vi "set channel.vi"(0 "VISA in":refnum<visa-resource-name>, 1 "Location Cluster in":T1, 2 "set row":i32, 3 "set card":i32, 4 "set channel":i32, 5 "error in":errorcluster) -> (14 "VISA out":refnum<visa-resource-name>, 15 "Location Cluster out":T1, 19 "error out":errorcluster)   [LabVIEW 2018]
uses:
  location cluster.ctl
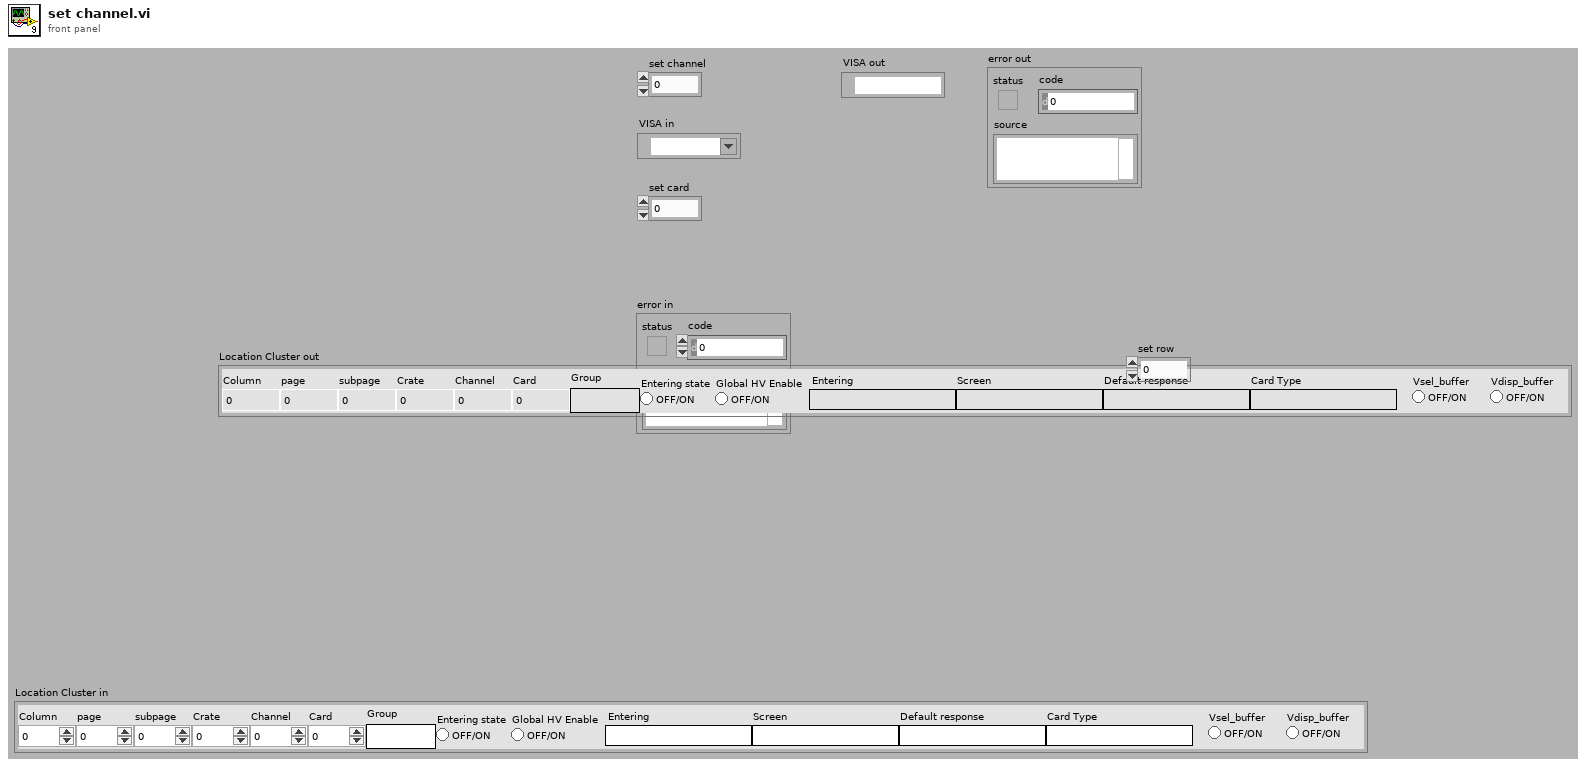
[diagram p1: front panel]
types:
  T1 = typedef "location cluster.ctl" = cluster{"Column":i32, "Card Type":string, "Channel":i32, "Card":i32, "Default response":string, "Entering":string, "Entering state":bool, "subpage":i32, "page":i32, "Crate":i32, "Screen":string, "Group":string, "Global HV Enable":bool, "Vsel_buffer":bool, "Vdisp_buffer":bool}
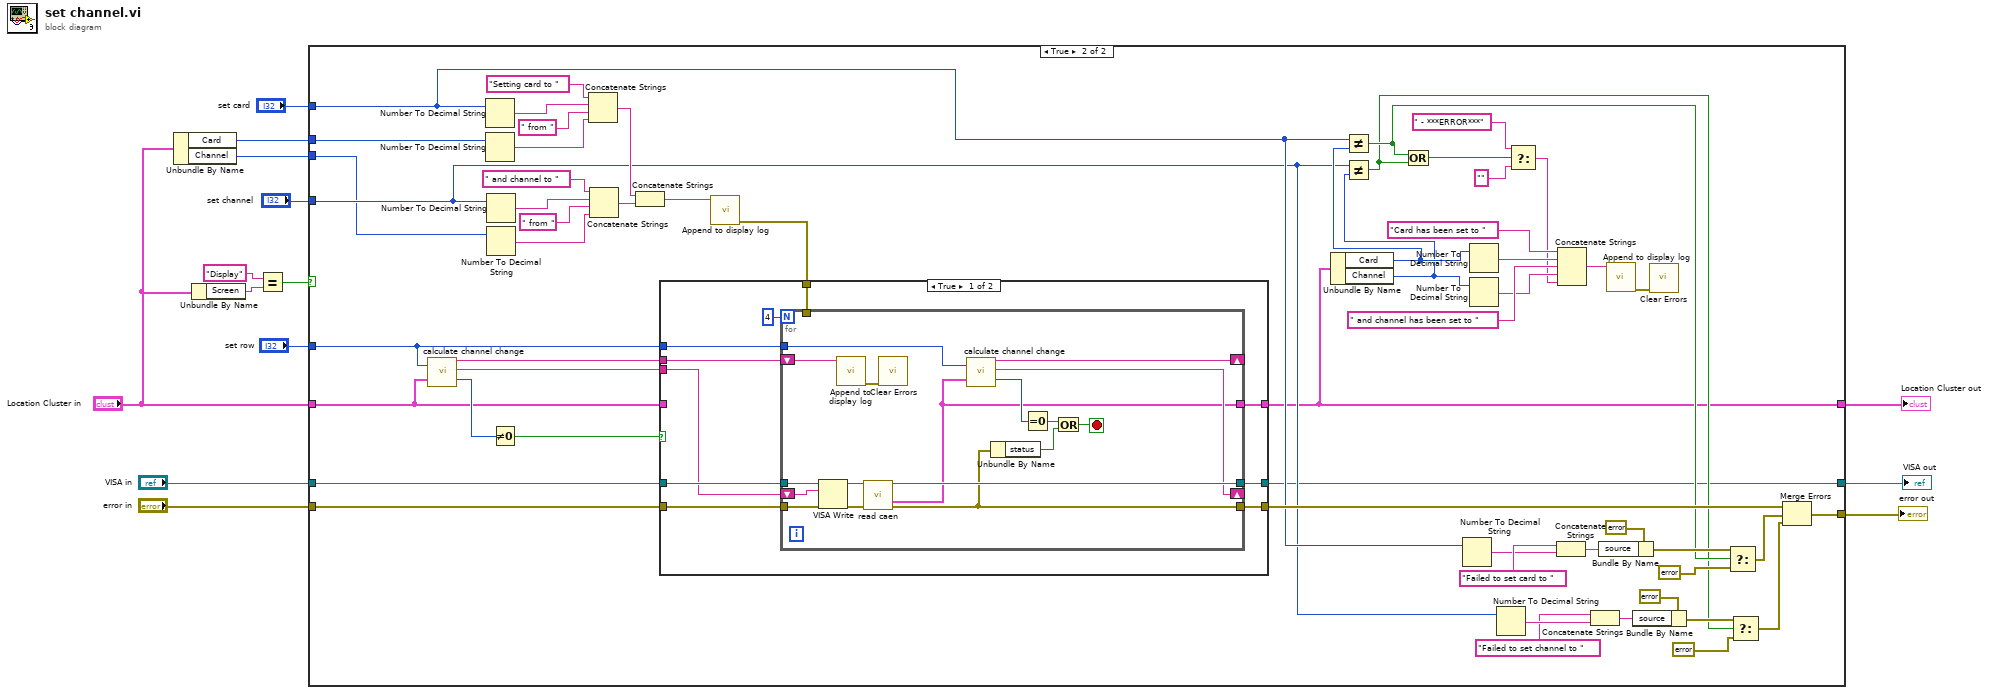
[diagram p0: block diagram]
diagram:
  n1 = Unbundle By Name("Location Cluster in") -> ("Card"=w9:i32, "Channel"=w2:i32)
  n2 = Unbundle By Name("Location Cluster in") -> ("Screen"=w12:string)
  n3 = Equal?(x="Display", y=w12) -> (x = y?=w5:bool)
  n4 = case shown="True" w5 {
    tunnel: "VISA in" -> [w16 w73]
    tunnel: "Location Cluster in" -> [w15 w18]
    tunnel: "error in" -> [w17 w19]
    tunnel: w9 -> [_ w48]
    tunnel: [w17 w36] -> w8
    tunnel: "set card" -> [_ w26]
    tunnel: "set channel" -> [_ w25]
    tunnel: w2 -> [_ w24]
    tunnel: [w15 w22] -> w4
    tunnel: [w16 w21] -> w3
    tunnel: "set row" -> [_ w20]
    frame False {
    }
    frame True {
      n5 = call "calculate channel change.vi"("set index"=w20, "Location Cluster in"=w18) -> ("action"=w46:string, "keystrokes"=w47:string, "rows difference"=w45:i32)  [unwired: 15 in]
      n6 = Number To Decimal String(number=w26) -> (decimal integer string=w66:string)  [unwired: 1 in]
      n7 = Number To Decimal String(number=w48) -> (decimal integer string=w68:string)  [unwired: 1 in]
      n8 = Number To Decimal String(number=w25) -> (decimal integer string=w71:string)  [unwired: 1 in]
      n9 = Number To Decimal String(number=w24) -> (decimal integer string=w69:string)  [unwired: 1 in]
      n10 = Not Equal To 0?(x=w45) -> (x != 0?=w23:bool)
      n11 = Concatenate Strings("Setting card to " ("string"), w66, " from " ("string"), w68) -> (w64:string)
      n12 = Concatenate Strings(" and channel to " ("string"), w71, " from " ("string"), w69) -> (w63:string)
      n13 = Concatenate Strings(w64, w63) -> (w62:string)
      n14 = call "Append to display log.vi"("string"=w62) -> ("error out"=w61:errorcluster)  [unwired: 10 in]
      n15 = case shown="True" w23 {
        tunnel: [w76 w103] -> w21
        tunnel: w73 -> [w83 w103]
        tunnel: [w82 w102] -> w37
        tunnel: w19 -> [w81 w102]
        tunnel: [w77 w101] -> w22
        tunnel: w18 -> [_ w101]
        tunnel: w61 -> [w74 _]
        tunnel: w20 -> [w80 _]
        tunnel: w47 -> [w78 _]
        tunnel: w46 -> [w79 _]
        frame True {
          n16 = for {
            N: 4 -> [_]
            tunnel: w80 -> [w95]
            tunnel: [w84] -> w77
            shift-right: [w86] -> _
            shift-left: w78 -> [w93]
            shift-right: [w85] -> _
            shift-left: w79 -> [w94]
            tunnel: w83 -> [w100]
            tunnel: [w91] -> w76
            tunnel: w81 -> [w97]
            tunnel: [w90] -> w82
            tunnel: w74 -> [_]
            stop <- w87 stop-if-true
            n17 = VISA Write(VISA resource name=w100, write buffer=w93, error in (no error)=w97) -> (VISA resource name out=w99:refnum<visa-resource-name>, error out=w98:errorcluster)  [unwired: 1 out]
            n18 = call "Append to display log.vi"("string"=w94) -> ("error out"=w92:errorcluster)  [unwired: 10 in]
            n19 = call "read caen.vi"("VISA in"=w99, "error in"=w98) -> ("VISA out"=w91:refnum<visa-resource-name>, "Location Cluster"=w84:T1, "error out"=w90:errorcluster)  [unwired: 8 in, 3 out]
            n20 = call <vilib>:"Clear Errors.vi"("error in (no error)"=w92) -> ()  [unwired: 5 in, 2 out]
            n21 = call "calculate channel change.vi"("set index"=w95, "Location Cluster in"=w84) -> ("action"=w85:string, "keystrokes"=w86:string, "rows difference"=w96:i32)  [unwired: 15 in]
            n22 = Unbundle By Name(w90) -> ("status"=w88:bool)
            n23 = Equal To 0?(x=w96) -> (x = 0?=w89:bool)
            n24 = Or(x=w89, y=w88) -> (x .or. y?=w87:bool)
          }
        }
        frame False {
        }
      }
      n25 = Unbundle By Name(w22) -> ("Card"=w50:i32, "Channel"=w49:i32)
      n26 = Not Equal?(x=w26, y=w50) -> (x != y?=w29:bool)
      n27 = Not Equal?(x=w25, y=w49) -> (x != y?=w28:bool)
      n28 = Or(x=w29, y=w28) -> (x .or. y?=w51:bool)
      n29 = Number To Decimal String(number=w26) -> (decimal integer string=w38:string)  [unwired: 1 in]
      n30 = Number To Decimal String(number=w50) -> (decimal integer string=w59:string)  [unwired: 1 in]
      n31 = Number To Decimal String(number=w49) -> (decimal integer string=w56:string)  [unwired: 1 in]
      n32 = Number To Decimal String(number=w25) -> (decimal integer string=w35:string)  [unwired: 1 in]
      n33 = Select(t=" - ***ERROR***" ("string"), s=w51, f="" ("string")) -> (s? t:f=w52:string)
      n34 = Concatenate Strings("Failed to set card to " ("string"), w38) -> (w40:string)
      n35 = Concatenate Strings("Card has been set to " ("string"), w59, " and channel has been set to " ("string"), w56, w52) -> (w57:string)
      n36 = Concatenate Strings("Failed to set channel to " ("string"), w35) -> (w33:string)
      n37 = Bundle By Name(cluster=errorcluster {"status"=TRUE, "code"=0, "source"=""} ("error in"), "source"=w40) -> (w41:errorcluster)
      n38 = call "Append to display log.vi"("string"=w57) -> ("error out"=w55:errorcluster)  [unwired: 10 in]
      n39 = Bundle By Name(cluster=errorcluster {"status"=TRUE, "code"=0, "source"=""} ("error in"), "source"=w33) -> (w32:errorcluster)
      n40 = call <vilib>:"Clear Errors.vi"("error in (no error)"=w55) -> ()  [unwired: 5 in, 2 out]
      n41 = Select(t=w41, s=w29, f=errorcluster {"status"=FALSE, "code"=0, "source"=""} ("error in")) -> (s? t:f=w44:errorcluster)
      n42 = Select(t=w32, s=w28, f=errorcluster {"status"=FALSE, "code"=0, "source"=""} ("error in")) -> (s? t:f=w27:errorcluster)
      n43 = Merge Errors(w37, w44, w27) -> (w36:errorcluster)
    }
  }
  "error out" <- w8
  "Location Cluster out" <- w4
  "VISA out" <- w3
